vi "Stop Core.vi"(10 "final error code":i32, 11 "Turbo in":refnum<class "Turbo.lvclass">) -> (3 "Turbo out":refnum<class "Turbo.lvclass">)   [LabVIEW 2015, in "cRIO-Carbondioxide.lvlib" / "CO2-Actor.lvlib" / "Turbo.lvclass"]
doc: "(<B>Filename</B>: Actor Framework.lvlib:Actor.lvclass:Stop Core.vi)\n\nDefines what the actor does before it stops. Use the <B>final error code</B> input to determine whether the actor shut down in response to an error.\n\nBy default, this method does nothing. A descendant class may override it to define behavior, such as shutting down any processes the actor initiated in its override of the Actor Core method."
uses:
  Turbo.lvclass
  <vilib>/ActorFramework/Time-Delayed Send Message/Time-Delay Override Options.ctl
  Turbo.lvclass/Turbo.ctl
  <vilib>/ActorFramework/Message Enqueuer/Message Enqueuer.lvclass/Message Enqueuer.ctl
  <vilib>/ActorFramework/Message Enqueuer/Enqueue.vi
  <vilib>/ActorFramework/Message Priority Queue/Priority Enqueue.vi
  <vilib>/ActorFramework/Stop Msg/Stop Msg.lvclass
  CO2 Actor/CO2 Actor.lvclass
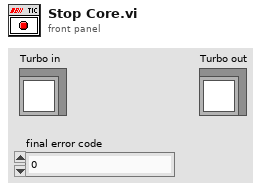
[diagram p1: front panel]
types:
  T1 = typedef "Time-Delay Override Options.ctl" = enum16{"Send next copy now", "Skip next scheduled copy", "Send next copy now and stop all further copies", "Stop all further copies"}
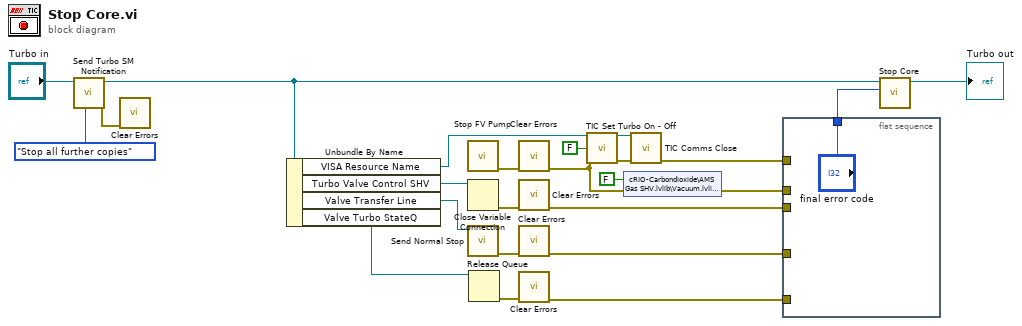
[diagram p0: block diagram]
diagram:
  n1 = call "Send Turbo SM Notification.vi"("notification (Send next copy now)"=Time-Delay_Override_Options."Stop all further copies", "Turbo in"="Turbo in") -> ("error out"=w18:errorcluster, "Turbo out"=w12:refnum<class "Turbo.lvclass">)  [unwired: 8 in]
  n2 = call <vilib>:"Clear Errors.vi"("error in (no error)"=w18) -> ()  [unwired: 5 in, 2 out]
  n3 = Unbundle By Name(w12) -> ("VISA Resource Name"=w7:refnum<visa-resource-name>, "Turbo Valve Control SHV"=w21:refnum<k21>, "Valve Transfer Line"=w15:refnum<class "Message Enqueuer.lvclass">, "Valve Turbo StateQ"=w14:refnum<queue>)
  n4 = call "Stop FV Pump.vi"() -> ("error out"=w5:errorcluster)  [unwired: 11 in]
  n5 = Close Variable Connection(11:w21) -> (0:w20:errorcluster)  [unwired: 1 in]
  n6 = call <vilib>:"Send Normal Stop.vi"("Message Enqueuer"=w15) -> ("error out"=w17:errorcluster)  [unwired: 10 in]
  n7 = Release Queue(queue=w14) -> (error out=w13:errorcluster)  [unwired: 2 in, 2 out]
  n8 = call <vilib>:"Clear Errors.vi"("error in (no error)"=w5) -> ("error out"=w3:errorcluster)  [unwired: 5 in, 1 out]
  n9 = call <vilib>:"Clear Errors.vi"("error in (no error)"=w20) -> ("error out"=w11:errorcluster)  [unwired: 5 in, 1 out]
  n10 = call <vilib>:"Clear Errors.vi"("error in (no error)"=w17) -> ("error out"=w10:errorcluster)  [unwired: 5 in, 1 out]
  n11 = call <vilib>:"Clear Errors.vi"("error in (no error)"=w13) -> ("error out"=w9:errorcluster)  [unwired: 5 in, 1 out]
  n12 = call <instrlib>:"TIC Set Turbo On - Off.vi"("VISA Session In"=w7, "On (F)"=FALSE, "error in (no error)"=w3) -> ("VISA Session (Dup)"=w6:refnum<visa-resource-name>, "error out"=w4:errorcluster)  [unwired: 11 in]
  n13 = shared-variable "cRIO-Carbondioxide\\AMS Gas SHV.lvlib\\Vacuum.lvlib\\Turbo ON"(FALSE ("Turbo ON"), error in=w3) -> (error out=w1:errorcluster)
  n14 = call <instrlib>:"TIC Comms Close.vi"("VISA Resource Name"=w6, "error in (no error)"=w4) -> ("error out"=w8:errorcluster)  [unwired: 13 in]
  n15 = flat-sequence {
    tunnel: ["final error code"] -> w23
    tunnel: w8 -> [_]
    tunnel: w11 -> [_]
    tunnel: w10 -> [_]
    tunnel: w9 -> [_]
    tunnel: w1 -> [_]
    frame #0 {
    }
  }
  n16 = call-parent "Stop Core.vi"("final error code"=w23, "CO2 Actor in"=w12) -> ("CO2 Actor out"=→"Turbo out":refnum<class "Turbo.lvclass">)  [unwired: 9 in]
